vi "Byte Buffer.Read (U32).vi"(8 "error in (no error)":errorcluster, 10 "buffer offset":i32, 11 "Byte Buffer in":refnum<class "Byte Buffer.lvclass">) -> (0 "error out":errorcluster, 1 "value":u32, 3 "Byte Buffer out":refnum<class "Byte Buffer.lvclass">)   [LabVIEW 2016, in "VeriStand Data.lvlib" / "Byte Buffer.lvclass"]
doc: "Reads one element of data from the provided <B>Byte Buffer</B> at location <B>buffer offset</B> in the format of the data type specified."
uses:
  Byte Buffer.lvclass
  Byte Buffer.lvclass/Byte Buffer.ctl
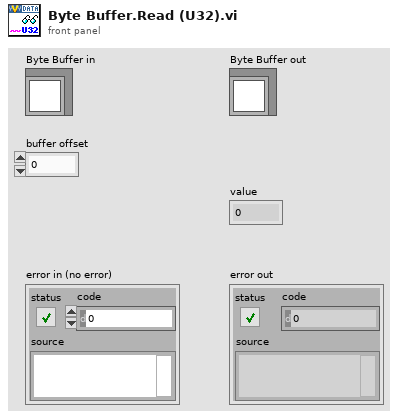
[diagram p1: front panel]
types:
  T1 = enum16{"big-endian, network order", "native, host order", "little-endian"}
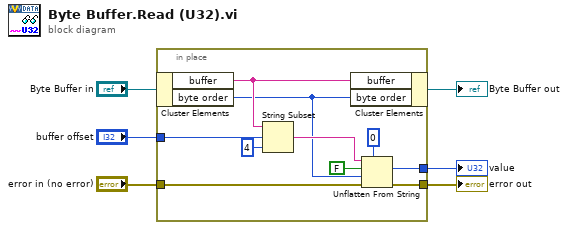
[diagram p0: block diagram]
diagram:
  n1 = in-place {
    in-place-border: "buffer offset" -> [w16]
    in-place-border: "error in (no error)" -> [w14]
    in-place-border: [w11] -> w4
    in-place-border: [w10] -> w3
    n2 = in-place-cluster #1("Byte Buffer in") -> ("buffer"=w9:string, "byte order"=w8:T1)
    n3 = String Subset(string=w9, offset (0)=w16, length (rest)=4 ("length (rest)")) -> (substring=w15:string)
    n4 = in-place-cluster #1("buffer"=w9, "byte order"=w8) -> (→"Byte Buffer out":refnum<class "Byte Buffer.lvclass">)
    n5 = Unflatten From String(type=u32 0, binary string=w15, data includes array or string size? (T)=FALSE, byte order (0:big-endian, network order)=w8, error in (no error)=w14) -> (value=w10:u32, error out=w11:errorcluster)  [unwired: 1 out]
  }
  "value" <- w3
  "error out" <- w4
